vi "NA Cluster v1_0_0.vi"() -> (0 "FVP  MAIN":T2={"general"={"project directory"=path "C:/NA", "User Name"="", "User Level"="", "valid login"=TRUE, "screen size"=1, "Screen Width"=1, "Screen Height"=1, "Login Password"="", "Login User Name"="", ".ini Resources"=[], "Control Refs"=[], "Error Ref out"=refnum}, "rendezvous"=refnum, "queues"={"Main"=refnum, "Error"=refnum, "VFP"=refnum, "STATUS"=refnum}, "NI Testand Config"={"NI_Teststand DB"=[]}, "Test Station Config"={"Test Station DB"=[], "Button Names"=[], "Short-cut keys"=[], "Paths to vis"=[], "Sub-Panel"=[], "Wait until done"=[], "Delay"=[], "Dispose Ref"=[], "Var. 1"=[], "Var. 2"=[], "Descriptions"=[], "Show Button"=[], "Short-cut from DB"=[], "Prefix"=[]}, "Sub Panel"={"Position"={"Left"=0, "Top"=0}, "Hidden Pos"={"Left"=0, "Top"=0}}, "Paths"={"Upload"=path "", "Processing"=path "", "Repository"=path "", "Finished"=path "", "Error"=path "", "Modelers"=path ""}, "Uploaded Jobs"=[], "Waiting Jobs"=[], "InProcess Jobs"=[], "Compute Engine"={"EXE"="", "Start Port"=0, "Execution Limit"=0, "Log"="", "Max Time Sec"=0.0}, "Computing Buffer"=[], "Slot Open?"=FALSE, "Retry"=0, "CPU Cores"="", "StatusBoard"=path "", "Retry Delay"=0.0})   [LabVIEW 2015]
doc: "WGLOV Cluster v1_0_0.vi\n\n\nGeneral Cluster constant used for start of state machine templates"
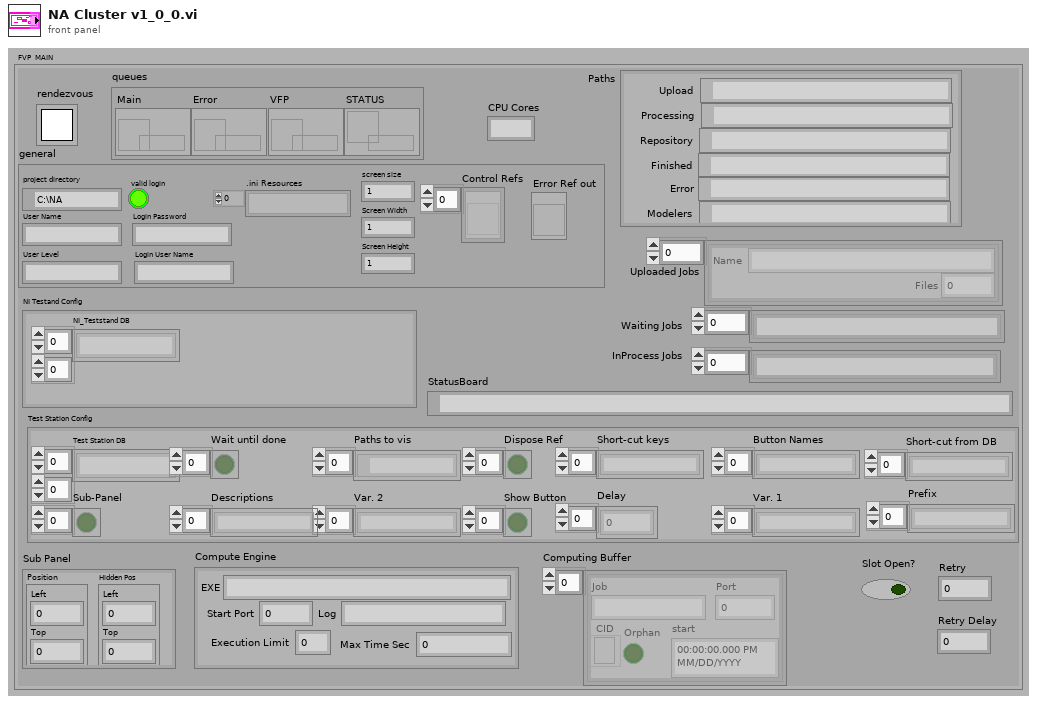
[diagram p1: front panel]
types:
  T1 = typedef "Rendezvous RefNum" = refnum<k1>
  T2 = cluster{"general":cluster{"project directory":path, "User Name":string, "User Level":string, "valid login":bool, "screen size":i32, "Screen Width":i32, "Screen Height":i32, "Login Password":string, "Login User Name":string, ".ini Resources":string[], "Control Refs":refnum<vi>[], "Error Ref out":refnum<vi>}, "rendezvous":T1, "queues":cluster{"Main":refnum<queue>, "Error":refnum<queue>, "VFP":refnum<queue>, "STATUS":refnum<queue>}, "NI Testand Config":cluster{"NI_Teststand DB":string[][]}, "Test Station Config":cluster{"Test Station DB":string[][], "Button Names":string[], "Short-cut keys":string[], "Paths to vis":path[], "Sub-Panel":bool[], "Wait until done":bool[], "Delay":i32[], "Dispose Ref":bool[], "Var. 1":string[], "Var. 2":string[], "Descriptions":string[], "Show Button":bool[], "Short-cut from DB":string[], "Prefix":string[]}, "Sub Panel":cluster{"Position":cluster{"Left":i32, "Top":i32}, "Hidden Pos":cluster{"Left":i32, "Top":i32}}, "Paths":cluster{"Upload":path, "Processing":path, "Repository":path, "Finished":path, "Error":path, "Modelers":path}, "Uploaded Jobs":cluster{"Name":string, "Files":i32}[], "Waiting Jobs":string[], "InProcess Jobs":string[], "Compute Engine":cluster{"EXE":string, "Start Port":i32, "Execution Limit":i32, "Log":string, "Max Time Sec":dbl}, "Computing Buffer":cluster{"Job":string, "Port":i32, "CID":refnum<k5>, "Orphan":bool, "start":timestamp}[], "Slot Open?":bool, "Retry":u32, "CPU Cores":string, "StatusBoard":path, "Retry Delay":dbl}
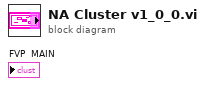
[diagram p0: block diagram]
diagram:
